vi "Get Stop Notifier Status.vi"(8 "error in (no error)":errorcluster, 11 "Sift Client in":refnum<class "Sift Client.lvclass">) -> (0 "error out":errorcluster, 2 "Fired":bool, 3 "Sift Client out":refnum<class "Sift Client.lvclass">)   [LabVIEW 2024, in "Sift Client.lvlib" / "Sift Client.lvclass"]
doc: "Returns True if the Stop Notifier was fired.\n\nUse this in any parallel loops to determine if they should stop queuing/writing data."
uses:
  Sift Client.lvclass
  Sift Client.lvclass/Sift Client.ctl
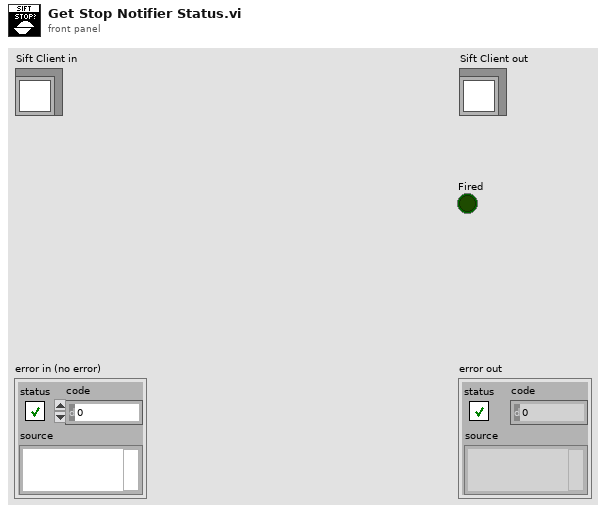
[diagram p1: front panel]
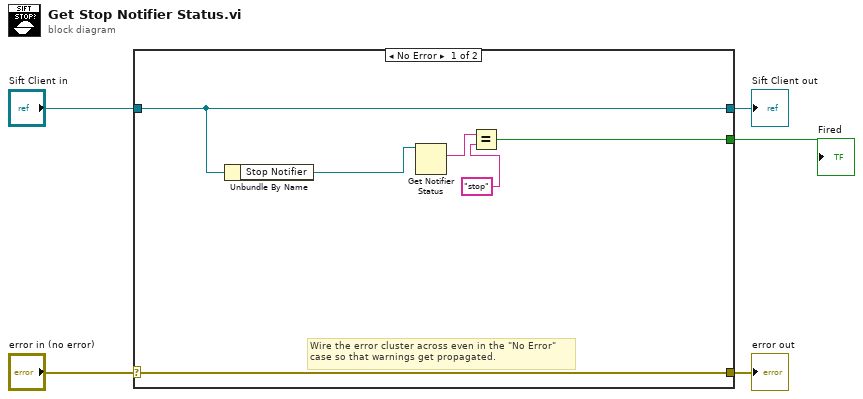
[diagram p0: block diagram]
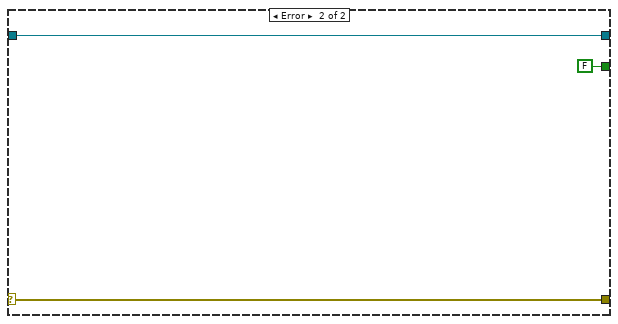
[diagram p2: hidden frame]
diagram:
  n1 = case shown="No Error" "error in (no error)" {
    selector: "error in (no error)" -> [w11 w14]
    tunnel: [w11 w14] -> w4
    tunnel: [w6 w13] -> w2
    tunnel: "Sift Client in" -> [w6 w13]
    tunnel: [w7 FALSE] -> w1
    frame No Error {
      # "Wire the error cluster across even in the \"No Error\"\ncase so that warnings get propagated."
      n2 = Unbundle By Name(w6) -> ("Stop Notifier"=w10:refnum<notifier>)
      n3 = Get Notifier Status(notifier=w10) -> (current notification=w9:string)  [unwired: 1 in, 4 out]
      n4 = Equal?(x=w9, y="stop") -> (x = y?=w7:bool)
    }
    frame Error {
    }
  }
  "error out" <- w4
  "Sift Client out" <- w2
  "Fired" <- w1
